vi "Close Notebook Window Action.vi"(8 "Notebook Saved?":bool, 9 "Main VI Name":string, 11 "Notebook Queue":refnum<queue>) -> (0 "Quit?":bool)   [LabVIEW 2021, in "Notebook.lvlib"]
uses:
  Notebook.lvlib
  Notebook Action Q Element.ctl
  Notebook Action List.ctl
  GUI/3-Button Dialog Output.ctl
  Fits/Fits.lvlib
  GUI/GUI.lvlib
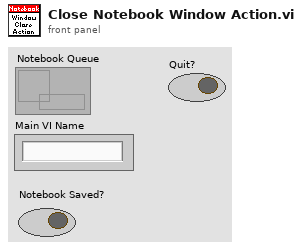
[diagram p1: front panel]
types:
  T1 = typedef "Fits.lvlib/3-Button Dialog Output.ctl" = enum16{"Window Close", "Button 1", "Button 2", "Button 3"}
  T2 = typedef "Notebook.lvlib/Notebook Action Q Element.ctl" = cluster{"Action":T3, "Variant":variant}
  T3 = typedef "Notebook.lvlib/Notebook Action List.ctl" = enum16{"Idle", "Init", "Check Content Change", "User added content", "Program added text", "Program added Picture ", "Save Notebook", "Quit", "Open", "Close", "Update Window Title"}
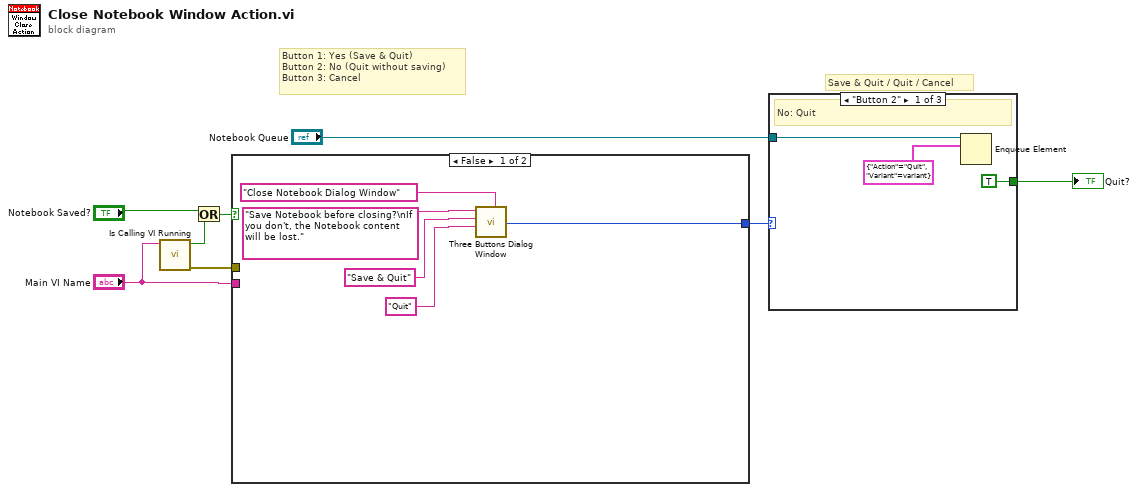
[diagram p0: block diagram]
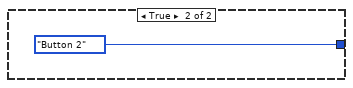
[diagram p2: hidden frame]
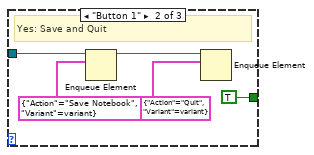
[diagram p3: hidden frame]
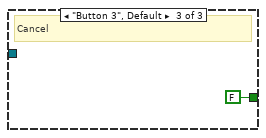
[diagram p4: hidden frame]
diagram:
  # "Button 1: Yes (Save & Quit)\nButton 2: No (Quit without saving)\nButton 3: Cancel"
  # "Save & Quit / Quit / Cancel"
  n1 = call "Is Calling VI Running.vi"("Calling VI Name"="Main VI Name") -> ("Error Out"=w1:errorcluster, "Running?"=w2:bool)  [unwired: 9 in]
  n2 = Or(x="Notebook Saved?", y=w2) -> (x .or. y?=w3:bool)
  n3 = case shown="False" w3 {
    tunnel: [w11 3-Button_Dialog_Output."Button 2" ("3-button Dialog Output")] -> w6
    tunnel: "Main VI Name" -> [_ _]
    tunnel: w1 -> [_ _]
    frame False {
      n4 = call "Three Buttons Dialog Window.vi"("Window Title"="Close Notebook Dialog Window" ("Window Title (\"\")"), "Button 2 Text"="Quit", "Button 1 Text (OK)"="Save & Quit", "Message"="Save Notebook before closing?\nIf you don't, the Notebook content will be lost." ("message")) -> ("3-button Dialog Output"=w11:T1)  [unwired: 7 in]
    }
    frame True {
    }
  }
  n5 = case shown="\"Button 2\"" w6 {
    tunnel: "Notebook Queue" -> [w17 w22 _]
    tunnel: [TRUE ("Discard?") TRUE ("Discard?") FALSE ("Discard?")] -> w7
    frame "Button 2" {
      # "No: Quit"
      n6 = Enqueue Element(queue=w17, element=T2 {"Action"=enum."Quit", "Variant"=variant}) -> ()  [unwired: 2 in, 3 out]
    }
    frame "Button 1" {
      # "Yes: Save and Quit"
      n7 = Enqueue Element(queue=w22, element=T2 {"Action"=enum."Save Notebook", "Variant"=variant}) -> (queue out=w20:refnum<queue>)  [unwired: 2 in, 2 out]
      n8 = Enqueue Element(queue=w20, element=T2 {"Action"=enum."Quit", "Variant"=variant}) -> ()  [unwired: 2 in, 3 out]
    }
    frame "Button 3", Default {
      # "Cancel"
    }
  }
  "Quit?" <- w7
